vi "alias_freq.vi"(9 "Fs":dbl, 11 "F":dbl) -> (3 "F aliased":dbl)   [LabVIEW 2012]
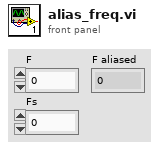
[diagram p1: front panel]
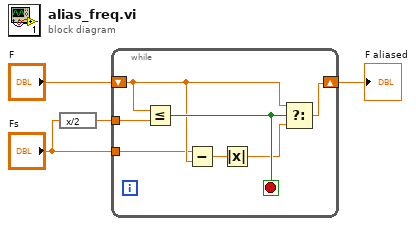
[diagram p0: block diagram]
diagram:
  n1 = expression code="x/2"("Fs") -> (w4:dbl)
  n2 = while {
    tunnel: w4 -> [w9]
    shift-right: [w10] -> w2
    shift-left: "F" -> [w8]
    tunnel: "Fs" -> [w5]
    stop <- w11 stop-if-true
    n3 = Less Or Equal?(x=w8, y=w9) -> (x <= y?=w11:bool)
    n4 = Subtract(x=w5, y=w8) -> (x-y=w7:dbl)
    n5 = Absolute Value(x=w7) -> (abs(x)=w6:dbl)
    n6 = Select(t=w8, s=w11, f=w6) -> (s? t:f=w10:dbl)
  }
  "F aliased" <- w2
